vi "follow the peak controller.vi"(7 "action":T2=enum."follow the peak", 11 "follow the peak ref":refnum<vi>) -> (1 "follow the peak OUT":T1={"factor"=3.0, "omega ?"=TRUE, "gamma ?"=TRUE, "max (kHz)"=3.0, "is clean"=TRUE, "acceptance"=0.3, "history - length"=10}, 3 "follow the peak ref OUT":refnum<vi>)   [LabVIEW 2015]
uses:
  follow the peak action.ctl
  follow the peak control.ctl
panel:
  in  "follow the peak":T1={"factor"=3.0, "omega ?"=TRUE, "gamma ?"=TRUE, "max (kHz)"=3.0, "is clean"=TRUE, "acceptance"=0.3, "history - length"=10}
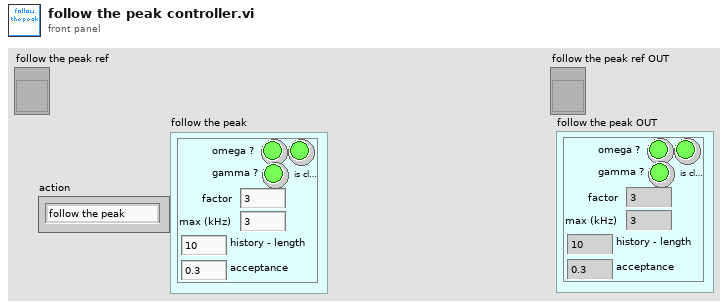
[diagram p1: front panel]
types:
  T1 = typedef "follow the peak control.ctl" = cluster{"factor":dbl, "omega ?":bool, "gamma ?":bool, "max (kHz)":dbl, "is clean":bool, "acceptance":dbl, "history - length":i32}
  T2 = typedef "follow the peak action.ctl" = enum16{"make clean", "make dirty", "follow the peak", "unfollow the peak", "follow gamma", "unfollow gamma", "check", "toggle omega", "toggle gamma"}
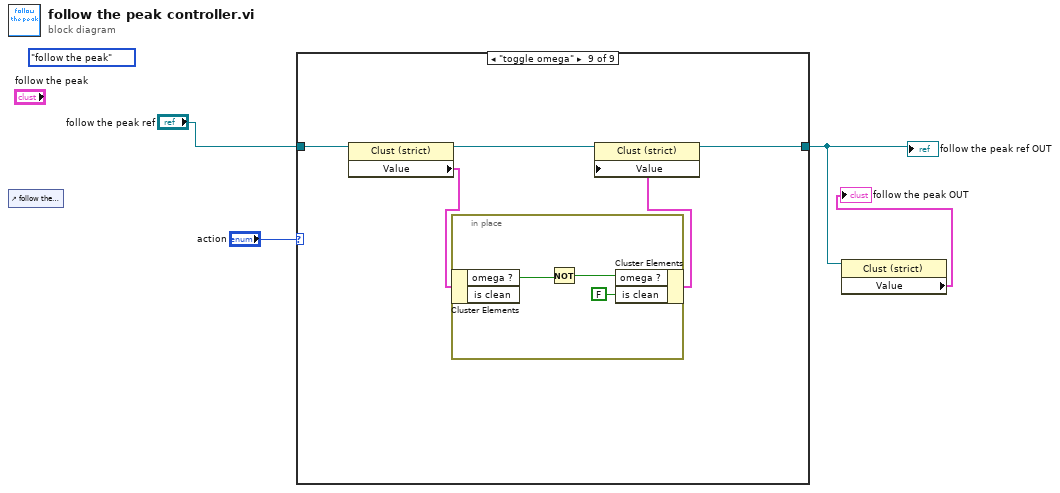
[diagram p0: block diagram]
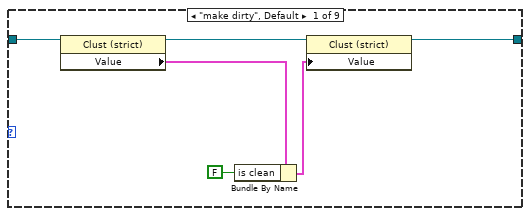
[diagram p2: hidden frame]
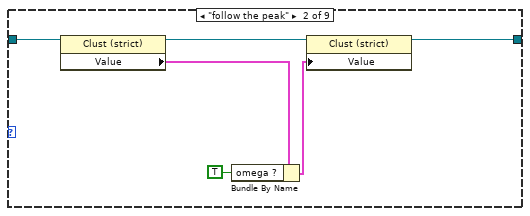
[diagram p3: hidden frame]
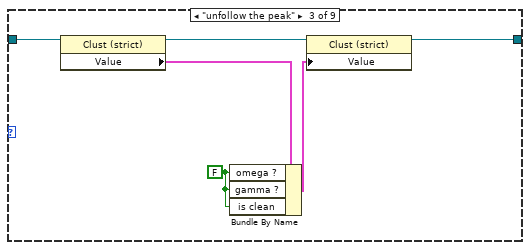
[diagram p4: hidden frame]
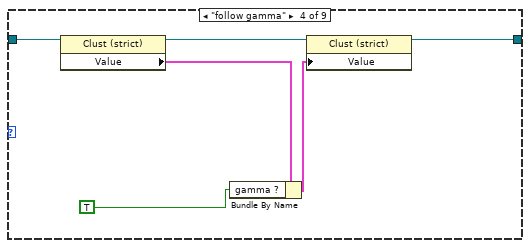
[diagram p5: hidden frame]
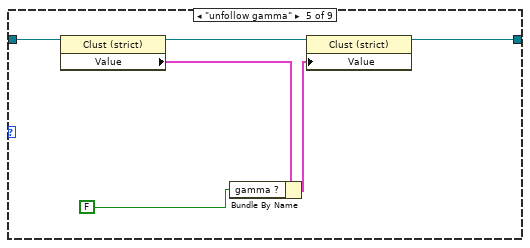
[diagram p6: hidden frame]
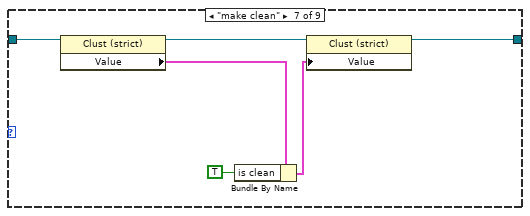
[diagram p8: hidden frame]
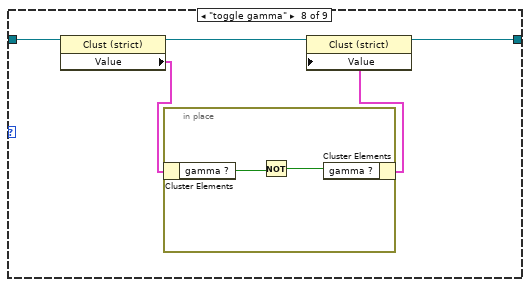
[diagram p9: hidden frame]
diagram:
  (unwired) follow_the_peak_action."follow the peak" ("action")
  n1 = control-ref of="follow the peak Con 2"() -> ()  [unwired: 1 out]
  n2 = case shown="\"toggle omega\"" "action" {
    tunnel: "follow the peak ref" -> [w10 w16 w22 w28 w34 w35 w41 w46 w53]
    tunnel: [w6 w12 w19 w25 w31 w35 w37 w44 w51] -> w2
    frame "make dirty", Default {
      n3 = property class="Clust (strict)"(reference=w10) -> (reference out=w7:refnum<vi>, "Value"=w9:T1)  [unwired: 1 in, 1 out]
      n4 = Bundle By Name(cluster=w9, "is clean"=FALSE ("omega ?")) -> (w5:T1)
      n5 = property class="Clust (strict)"(reference=w7, "Value"=w5) -> (reference out=w6:refnum<vi>)  [unwired: 1 in, 1 out]
    }
    frame "follow the peak" {
      n6 = property class="Clust (strict)"(reference=w16) -> (reference out=w13:refnum<vi>, "Value"=w15:T1)  [unwired: 1 in, 1 out]
      n7 = Bundle By Name(cluster=w15, "omega ?"=TRUE) -> (w11:T1)
      n8 = property class="Clust (strict)"(reference=w13, "Value"=w11) -> (reference out=w12:refnum<vi>)  [unwired: 1 in, 1 out]
    }
    frame "unfollow the peak" {
      w17 = FALSE ("omega ?")
      n9 = property class="Clust (strict)"(reference=w22) -> (reference out=w20:refnum<vi>, "Value"=w21:T1)  [unwired: 1 in, 1 out]
      n10 = Bundle By Name(cluster=w21, "omega ?"=w17, "gamma ?"=w17, "is clean"=w17) -> (w18:T1)
      n11 = property class="Clust (strict)"(reference=w20, "Value"=w18) -> (reference out=w19:refnum<vi>)  [unwired: 1 in, 1 out]
    }
    frame "follow gamma" {
      n12 = property class="Clust (strict)"(reference=w28) -> (reference out=w26:refnum<vi>, "Value"=w27:T1)  [unwired: 1 in, 1 out]
      n13 = Bundle By Name(cluster=w27, "gamma ?"=TRUE ("omega ?")) -> (w24:T1)
      n14 = property class="Clust (strict)"(reference=w26, "Value"=w24) -> (reference out=w25:refnum<vi>)  [unwired: 1 in, 1 out]
    }
    frame "unfollow gamma" {
      n15 = property class="Clust (strict)"(reference=w34) -> (reference out=w32:refnum<vi>, "Value"=w33:T1)  [unwired: 1 in, 1 out]
      n16 = Bundle By Name(cluster=w33, "gamma ?"=FALSE ("omega ?")) -> (w30:T1)
      n17 = property class="Clust (strict)"(reference=w32, "Value"=w30) -> (reference out=w31:refnum<vi>)  [unwired: 1 in, 1 out]
    }
    frame "check" {
    }
    frame "make clean" {
      n18 = property class="Clust (strict)"(reference=w41) -> (reference out=w38:refnum<vi>, "Value"=w40:T1)  [unwired: 1 in, 1 out]
      n19 = Bundle By Name(cluster=w40, "is clean"=TRUE ("omega ?")) -> (w36:T1)
      n20 = property class="Clust (strict)"(reference=w38, "Value"=w36) -> (reference out=w37:refnum<vi>)  [unwired: 1 in, 1 out]
    }
    frame "toggle gamma" {
      n21 = property class="Clust (strict)"(reference=w46) -> (reference out=w45:refnum<vi>, "Value"=w43:T1)  [unwired: 1 in, 1 out]
      n22 = in-place {
        n23 = in-place-cluster #1(w43) -> ("gamma ?"=w48:bool)
        n24 = Not(x=w48) -> (.not. x?=w47:bool)
        n25 = in-place-cluster #1("gamma ?"=w47) -> (w42:T1)
      }
      n26 = property class="Clust (strict)"(reference=w45, "Value"=w42) -> (reference out=w44:refnum<vi>)  [unwired: 1 in, 1 out]
    }
    frame "toggle omega" {
      n27 = property class="Clust (strict)"(reference=w53) -> (reference out=w52:refnum<vi>, "Value"=w50:T1)  [unwired: 1 in, 1 out]
      n28 = in-place {
        n29 = in-place-cluster #2(w50) -> ("omega ?"=w56:bool)  [unwired: 1 out]
        n30 = Not(x=w56) -> (.not. x?=w55:bool)
        n31 = in-place-cluster #2("omega ?"=w55, "is clean"=FALSE) -> (w49:T1)
      }
      n32 = property class="Clust (strict)"(reference=w52, "Value"=w49) -> (reference out=w51:refnum<vi>)  [unwired: 1 in, 1 out]
    }
  }
  "follow the peak ref OUT" <- w2
  n33 = property class="Clust (strict)"(reference=w2) -> ("Value"=→"follow the peak OUT":T1)  [unwired: 1 in, 2 out]
